vi "Get Port.vi"(8 "error in (no error)":errorcluster, 11 "Instrument.SR7270 in":refnum<class "Instrument.SR7270.lvclass">) -> (0 "error out":errorcluster, 2 "port":u32, 3 "Instrument.SR7270 out":refnum<class "Instrument.SR7270.lvclass">)   [LabVIEW 2016, in "Instrument.SR7270.lvclass"]
uses:
  Instrument.SR7270.lvclass
  levylab_inst/lvsrc/SMOs/Instrument/Instrument.lvclass
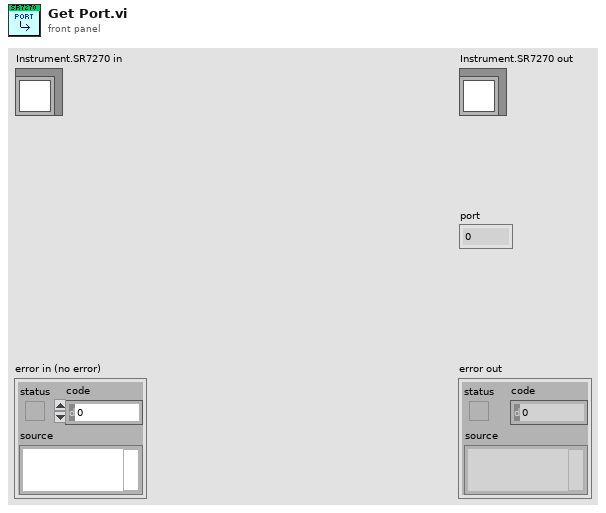
[diagram p1: front panel]
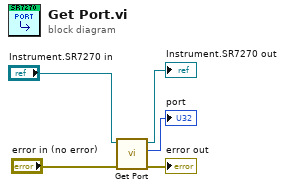
[diagram p0: block diagram]
diagram:
  n1 = call-parent "Get Port.vi"("error in (no error)"="error in (no error)", "Instrument in"="Instrument.SR7270 in") -> ("error out"=→"error out":errorcluster, "port"=→"port":u32, "Instrument out"=→"Instrument.SR7270 out":refnum<class "Instrument.SR7270.lvclass">)  [unwired: 7 in]
